vi "mqttCmdBuildVarHdr.vi"(0 "_mqtt in":refnum<class "mqttCmdPublish.lvclass">, 11 "error in (no error)":errorcluster) -> (4 "_mqtt out":refnum<class "mqttCmdPublish.lvclass">, 8 "variableHeader":u8[](array[numeric]) format="%02x", 15 "error out":errorcluster)   [LabVIEW 2020, in "mqttCmdPublish.lvclass"]
uses:
  mqttCmdPublish.lvclass
  C:/Projects/Libraries/Gore SM 2020/mqtt-LabVIEW/src/class/mqtt/mqttCmd/mqttCmd.lvclass
  mqttCmdPublish.lvclass/mqttCmdPublish.ctl
  mqttCmd.lvclass/mqttCmd.ctl
  Properties/Read QoS.vi
  Properties/Read messageID.vi
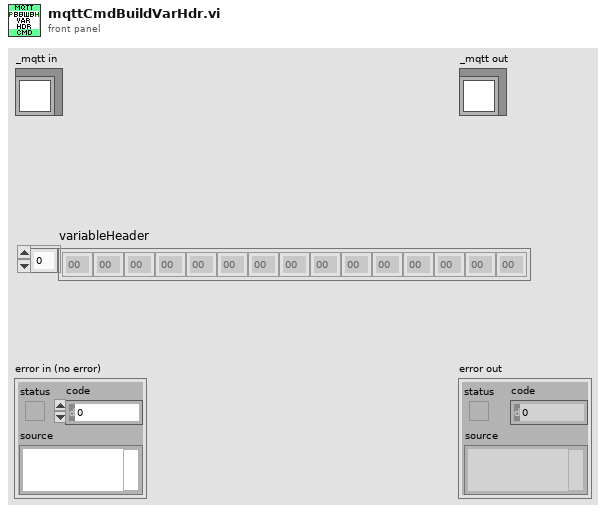
[diagram p1: front panel]
types:
  T1 = typedef "mqttQOSlevel.ctl" = enum8{"At most once", "At least once", "Exactly once", "Reserved"}
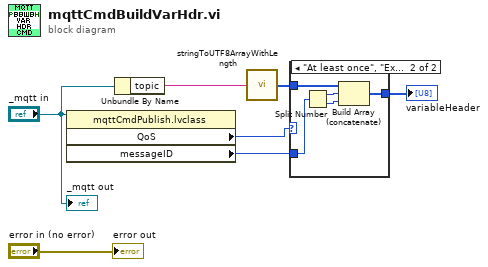
[diagram p0: block diagram]
diagram:
  n1 = property class="mqttCmdPublish.lvclass"(reference="_mqtt in") -> ("QoS"=w3:T1, "messageID"=w1:u16)  [unwired: 1 in, 2 out]
  n2 = Unbundle By Name("_mqtt in") -> ("topic"=w2:string)
  n3 = call "stringToUTF8ArrayWithLength.vi"("string"=w2) -> ("UTF8[]"=w6:u8[])  [unwired: 14 in]
  n4 = case shown="\"At least once\", \"Exactly once\"" w3 {
    tunnel: w1 -> [_ w11]
    tunnel: [w8 w10] -> w7
    tunnel: w6 -> [w8 w9]
    frame "At most once", Default {
    }
    frame "At least once", "Exactly once" {
      n5 = Split Number(x=w11) -> (hi(x)=w12:u8, lo(x)=w13:u8)
      n6 = Build Array (concatenate)(w9, w12, w13) -> (w10:u8[])
    }
  }
  "variableHeader" <- w7
  "error out" <- "error in (no error)"
  "_mqtt out" <- "_mqtt in"
